vi "RemoveEndOfLine.vi"(8 "error in":errorcluster, 11 "reboot log text":string) -> (0 "error out":errorcluster, 3 "reboot log text out":string)   [LabVIEW 2017]
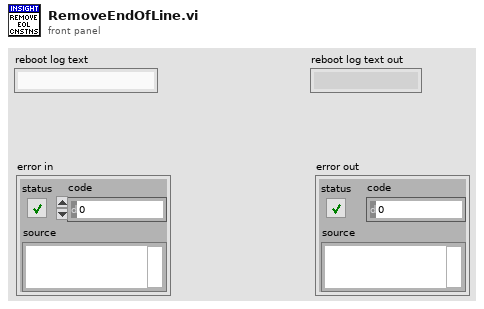
[diagram p1: front panel]
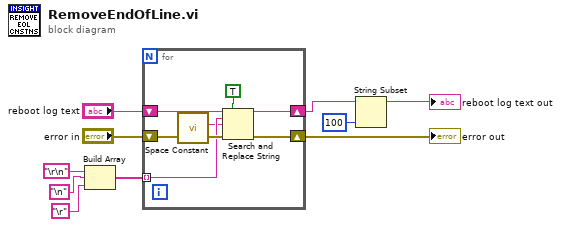
[diagram p0: block diagram]
diagram:
  n1 = Build Array("\r\n", "\n", "\r") -> (w6:string[])
  n2 = for {
    tunnel: w6 -> [w15] mode=indexing
    shift-right: [w13] -> w7
    shift-left: "reboot log text" -> [w16]
    shift-right: [w11] -> w3
    shift-left: "error in" -> [w17]
    n3 = call <vilib>:"Space Constant.vi"() -> ("String"=w14:string)
    n4 = Search and Replace String(replace all?=TRUE ("replace all? (F)"), input string=w16, search string=w15, replace string=w14, error in=w17) -> (result string=w13:string, error out=w11:errorcluster)  [unwired: 3 in, 2 out]
  }
  "error out" <- w3
  n5 = String Subset(string=w7, length (rest)=100 ("length (rest)")) -> (substring=→"reboot log text out":string)  [unwired: 1 in]
